vi "HealthCheckUI.vi"(10 "Edit Table":bool, 11 "Table in":refnum<vi>) -> ()   [LabVIEW 2018, in "HealthCheck.lvclass"]
uses:
  HealthCheck.lvclass
  HCState_TypeDef.ctl
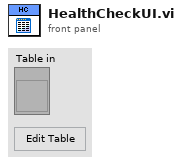
[diagram p1: front panel]
types:
  T1 = typedef "HealthCheck.lvclass/HCState_TypeDef.ctl" = enum16{"Initialization", "Running", "Modify Table"}
  T2 = enum32{"Invalid", "Standard", "Closed", "Hidden", "Minimized", "Maximized"}
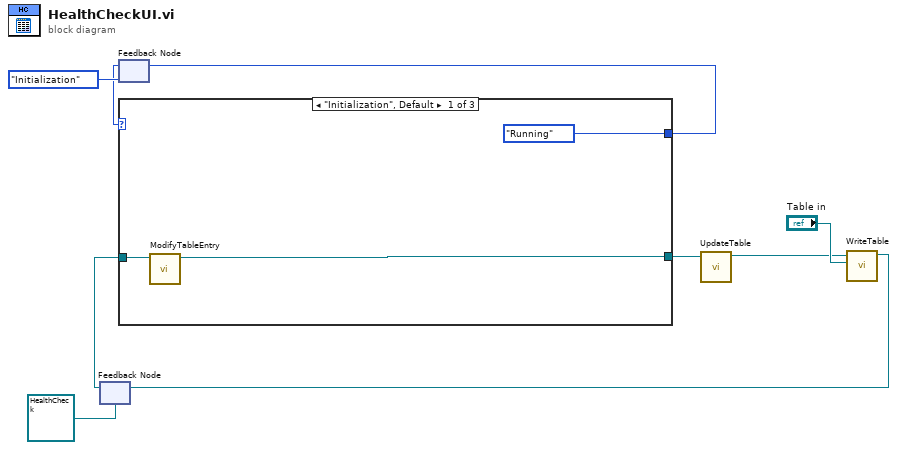
[diagram p0: block diagram]
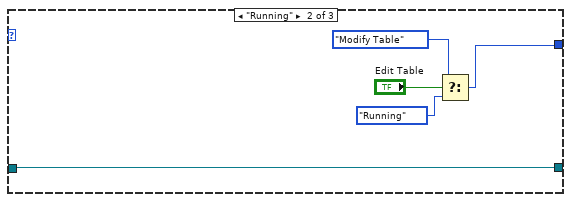
[diagram p2: hidden frame]
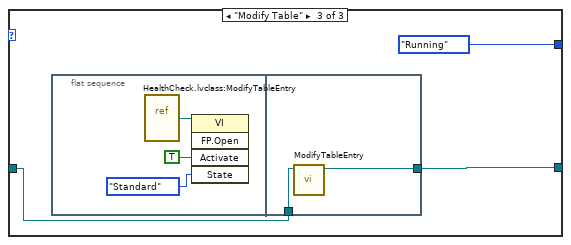
[diagram p3: hidden frame]
diagram:
  n1 = feedback #1(refnum<class "HealthCheck.lvclass"> refnum ("HealthCheck.lvclass")) -> (w5:refnum<class "HealthCheck.lvclass">)
  n2 = feedback #2(HCState_TypeDef."Initialization") -> (w8:T1)
  n3 = case shown="\"Initialization\", Default" w8 {
    tunnel: [HCState_TypeDef."Running" w17 HCState_TypeDef."Running"] -> w7
    tunnel: [w11 w13 w18] -> w2
    tunnel: w5 -> [w10 w13 w19]
    frame "Initialization", Default {
      n4 = call "ModifyTableEntry.vi"("HealthCheck in"=w10) -> ("HealthCheck out"=w11:refnum<class "HealthCheck.lvclass">)  [unwired: 9 in, 1 out]
    }
    frame "Running" {
      n5 = Select(t=HCState_TypeDef."Modify Table", s="Edit Table", f=HCState_TypeDef."Running") -> (s? t:f=w17:T1)
    }
    frame "Modify Table" {
      n6 = flat-sequence {
        tunnel: w19 -> [w25]
        tunnel: [w24] -> w18
        frame #0 {
          n7 = vi-ref "HealthCheck.lvclass:ModifyTableEntry.vi"() -> (w23:refnum<vi>)
          n8 = invoke class="VI" method="FP.Open"(reference=w23, "Activate"=TRUE ("Activate?"), "State"=T2."Standard") -> ()  [unwired: 2 in, 5 out]
        }
        frame #1 {
          n9 = call "ModifyTableEntry.vi"("HealthCheck in"=w25) -> ("HealthCheck out"=w24:refnum<class "HealthCheck.lvclass">)  [unwired: 9 in, 1 out]
        }
      }
    }
  }
  n10 = feedback-in #2(w7) -> ()
  n11 = call "UpdateTable.vi"("HealthCheck in"=w2) -> ("HealthCheck out"=w1:refnum<class "HealthCheck.lvclass">)  [unwired: 9 in, 1 out]
  n12 = call "WriteTable.vi"("Table in"="Table in", "HealthCheck in"=w1) -> ("HealthCheck out"=w4:refnum<class "HealthCheck.lvclass">)  [unwired: 8 in, 1 out]
  n13 = feedback-in #1(w4) -> ()
